vi "Close Variable Connections.vi"(11 "Variable References":T1) -> ()   [LabVIEW 2020]
uses:
  controls/Variable References.ctl
  controls/Raw Values.ctl
  controls/FPGA State.ctl
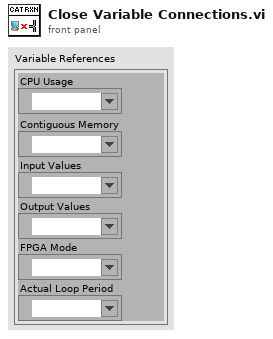
[diagram p1: front panel]
types:
  T1 = typedef "Variable References.ctl" = cluster{"CPU Usage":refnum<k21>, "Contiguous Memory":refnum<k21>, "Input Values":refnum<k21>, "Output Values":refnum<k21>, "FPGA Mode":refnum<k21>, "Actual Loop Period":refnum<k21>}
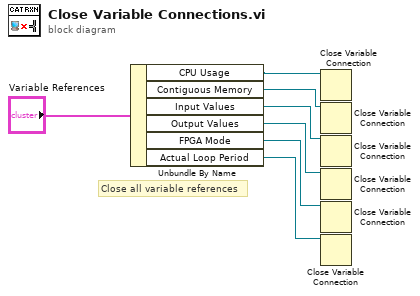
[diagram p0: block diagram]
diagram:
  # "Close all variable references"
  n1 = Unbundle By Name("Variable References") -> ("CPU Usage"=w2:refnum<k21>, "Contiguous Memory"=w3:refnum<k21>, "Input Values"=w4:refnum<k21>, "Output Values"=w5:refnum<k21>, "FPGA Mode"=w6:refnum<k21>, "Actual Loop Period"=w7:refnum<k21>)
  n2 = Close Variable Connection(11:w2) -> ()  [unwired: 1 in, 1 out]
  n3 = Close Variable Connection(11:w3) -> ()  [unwired: 1 in, 1 out]
  n4 = Close Variable Connection(11:w4) -> ()  [unwired: 1 in, 1 out]
  n5 = Close Variable Connection(11:w5) -> ()  [unwired: 1 in, 1 out]
  n6 = Close Variable Connection(11:w6) -> ()  [unwired: 1 in, 1 out]
  n7 = Close Variable Connection(11:w7) -> ()  [unwired: 1 in, 1 out]
